vi "SS2 Live_Init FPGA.vi"(6 "Live Mode":bool, 8 "Error In":errorcluster, 9 "Current Image Set":i32, 10 "FPGA bitfile Path":path=path "C:/Data on Delator/SwissSPAD2/Software  64bit/matlab_code_fast_var_gate_v2/bit_file/ss2_top.bit", 11 "SS2 Live Internal Variables in":T1={"okCFrontPanelDevices Refnum"=refnum, "Device Refnum"=refnum, "Display Image"=refnum, "# Live Images"=0, "relative s"=0.0, "# Image Sets"=0, "Message"="", "Current Image Set"=0, "# Datasets"=0, "Current Dataset"=0, "Live Mode"=FALSE, "Recording Mode"=FALSE, "Record Button"=refnum, "Live Button"=refnum, "SS2 Live Gate Data Q Name"="SS2 Live Gate Data Q", "Discard First Image"=FALSE, "Image Information"={"Save ROI Only"=FALSE, "Left"=0, "Top"=0, "Right"=0, "Bottom"=0, "Use Current ROI"=FALSE}, "Image Binning Options"={"Use Image Binning"=FALSE, "X Bin"=1, "Y Bin"=1}} {"Image Binning Options"."Y Bin" min=1; "Image Binning Options"."X Bin" min=1}) -> (0 "Error Out":errorcluster, 1 "# 8-bit Images per Set":u32, 2 "Buffer Size (#8-bit Images)":u32, 3 "SS2 Live Internal Variables out":T1={"okCFrontPanelDevices Refnum"=refnum, "Device Refnum"=refnum, "Display Image"=refnum, "# Live Images"=0, "relative s"=0.0, "# Image Sets"=0, "Message"="", "Current Image Set"=0, "# Datasets"=0, "Current Dataset"=0, "Live Mode"=FALSE, "Recording Mode"=FALSE, "Record Button"=refnum, "Live Button"=refnum, "SS2 Live Gate Data Q Name"="SS2 Live Gate Data Q", "Discard First Image"=FALSE, "Image Information"={"Save ROI Only"=FALSE, "Left"=0, "Top"=0, "Right"=0, "Bottom"=0, "Use Current ROI"=FALSE}, "Image Binning Options"={"Use Image Binning"=FALSE, "X Bin"=1, "Y Bin"=1}} {"Image Binning Options"."Y Bin" min=1; "Image Binning Options"."X Bin" min=1})   [LabVIEW 2019]
uses:
  SS2 Live Internal Variables.ctl
  C:/UCLA Thinkpad Google Drive/LabVIEW 2019 SP1/builds/SS2 Live Distribution/Opal Kelly/C# Wrapper/libFrontPanel-csharp.dll
  Opal Kelly/C# Wrapper/libFrontPanel-csharp.dll
  <vilib>/vision/Image Controls.llb/IMAQ Image.ctl
  SS2 Live_Image ROI Information.ctl
  Phasor/Image Binning Options.ctl
  SS2 Live_Settings List.ctl
  Opal Kelly/C# Wrapper/okFrontPanelC#Wrapper.lvlib
  Variant/Variant to Data/Variant to Data.lvlib
panel:
  in  "milliseconds to wait":u32
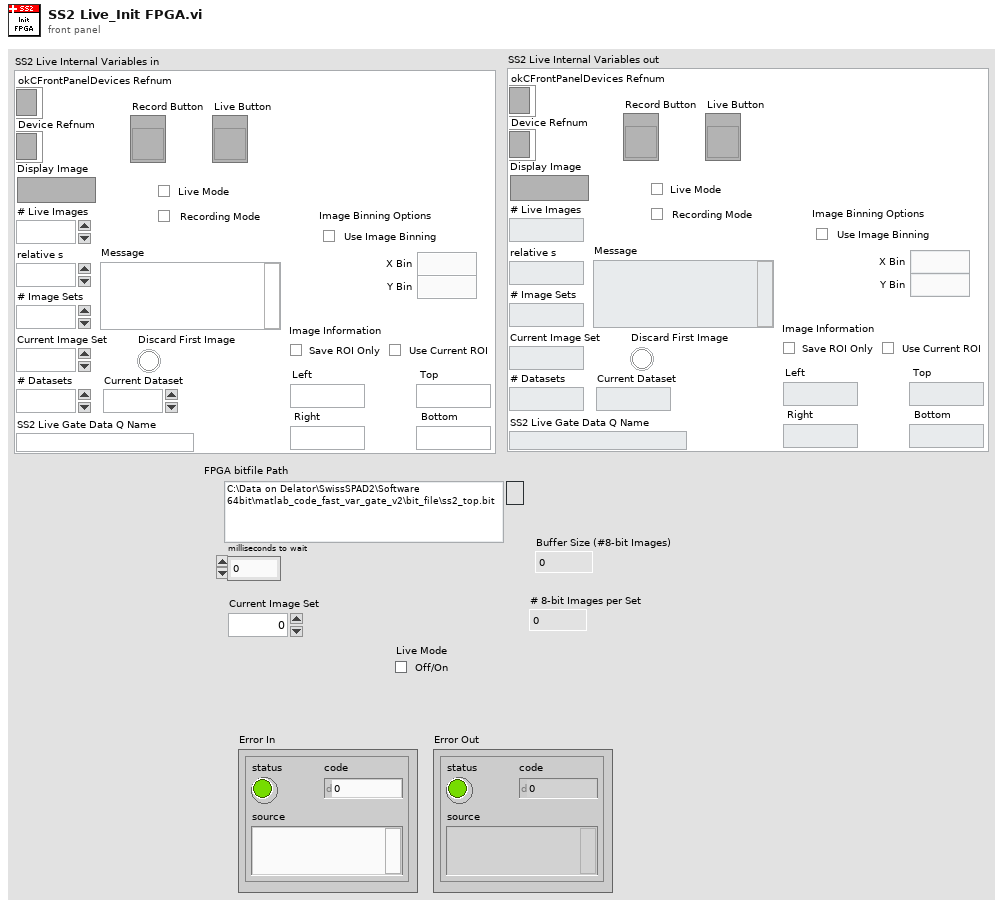
[diagram p1: front panel]
types:
  T1 = typedef "SS2 Live Internal Variables.ctl" = cluster{"okCFrontPanelDevices Refnum":refnum<k24>, "Device Refnum":refnum<k24>, "Display Image":T2, "# Live Images":i32, "relative s":dbl, "# Image Sets":i32, "Message":string, "Current Image Set":i32, "# Datasets":i32, "Current Dataset":i32, "Live Mode":bool, "Recording Mode":bool, "Record Button":refnum<vi>, "Live Button":refnum<vi>, "SS2 Live Gate Data Q Name":string, "Discard First Image":bool, "Image Information":T3, "Image Binning Options":T4}
  T2 = typedef "IMAQ Image.ctl" = refnum<image>
  T3 = typedef "SS2 Live_Image ROI Information.ctl" = cluster{"Save ROI Only":bool, "Left":u16, "Top":u16, "Right":u16, "Bottom":u16, "Use Current ROI":bool}
  T4 = typedef "Image Binning Options.ctl" = cluster{"Use Image Binning":bool, "X Bin":i32, "Y Bin":i32}
  T5 = typedef "SS2 Live_Settings List.ctl" = enum16{"FPGA:Bitfile Path", "FPGA:Bitfile Version", "Acquisition Parameters:SS2 DAQ Parameters", "Acquisition Parameters:Gate Configuration Array", "Acquisition Parameters:Buffer Size (# Gates)", "File Information:File Information", "File Information:# Datasets in Series", "Image Parameters:Image ROI Information", "Image Parameters:Image Binning Options", "UI Parameters:Histogram Bins Number"}
  T6 = typedef "SS2 DAQ Parameters 2.ctl" = cluster{"10 bits":bool, "# Exposure Sequences":u32, "# 1-bit Frame per Gate":u32, "Gate Shift":u32, "# Gates per Set":u32, "# Sets":u32, "Laser Period":dbl[unit], "Gate Offset":u32, "Auto-adjust Gate Offset":bool, "Gate Definition":T7}
  T7 = typedef "SS2 Gate Definition.ctl" = cluster{"gs_psincdec_0":u32, "gs_psincdec_1":u32, "gs_psincdec_2":u32, "gs_psincdec_3":u32, "gs_no_shift_adj_1":u32, "gs_no_shift_adj_2":u32, "gs_no_shift_adj_3":u32}
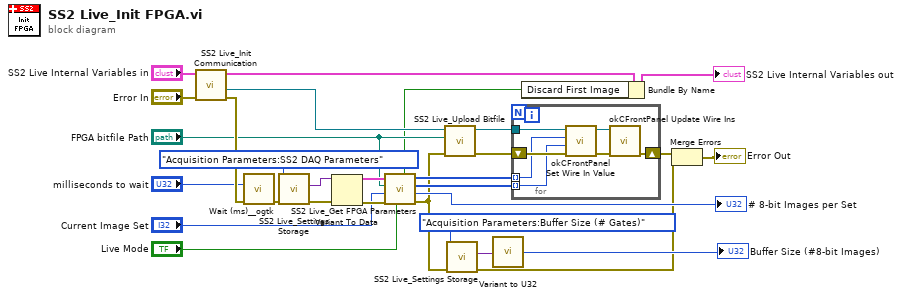
[diagram p0: block diagram]
diagram:
  n1 = call "SS2 Live_Init Communication.vi"("Error In"="Error In", "SS2 Live Internal Variables in"="SS2 Live Internal Variables in") -> ("Error Out"=w23:errorcluster, "Device Refnum"=w10:refnum<k24>, "SS2 Live Internal Variables out"=w9:T1)  [unwired: 6 in, 1 out]
  n2 = call <userlib>:"Wait (ms)__ogtk.vi"("error in (no error)"=w23, "milliseconds to wait"="milliseconds to wait") -> ("error out"=w13:errorcluster)  [unwired: 8 in, 1 out]
  n3 = call "SS2 Live_Settings Storage.vi"("Error In"=w13, "Settings List"=SS2_Live_Settings_List."Acquisition Parameters:SS2 DAQ Parameters") -> ("Error Out"=w20:errorcluster, "Variant Data out"=w21:variant)  [unwired: 8 in]
  n4 = Variant To Data(error in=w20, Variant=w21) -> (data=w17:T6, error out=w19:errorcluster)  [unwired: 1 in]
  n5 = call "SS2 Live_Get FPGA Parameters.vi"("Live Mode"="Live Mode", "Error In"=w19, "Current Image Set"="Current Image Set", "Bifile Path"="FPGA bitfile Path", "SS2 DAQ Parameters"=w17) -> ("Error Out"=w6:errorcluster, "#8-bit Images per Set"=→"# 8-bit Images per Set":u32, "SS2 FPGA DAQ Parameters"=w25:u32[], "SS2 FPGA DAQ Addresses"=w24:i32[], "Discard First Image"=w7:bool)  [unwired: 2 in]
  n6 = call "SS2 Live_Upload Bitfile.vi"("error in (no error)"=w6, "FPGA bitfile Path"="FPGA bitfile Path", "okCFrontPanel Device Refnum"=w10) -> ("error out"=w28:errorcluster, "okCFrontPanel Device Refnum"=w27:refnum<k24>)  [unwired: 7 in]
  n7 = call "SS2 Live_Settings Storage.vi"("Error In"=w6, "Settings List"=SS2_Live_Settings_List."Acquisition Parameters:Buffer Size (# Gates)") -> ("Error Out"=w1:errorcluster, "Variant Data out"=w4:variant)  [unwired: 8 in]
  n8 = call "Variant to U32.vi"("Variant"=w4) -> ("Value"=→"Buffer Size (#8-bit Images)":u32)  [unwired: 8 in]
  n9 = for {
    shift-right: [w31] -> w26
    shift-left: w28 -> [w36]
    tunnel: w25 -> [w34] mode=indexing
    tunnel: w24 -> [w30] mode=indexing
    tunnel: w27 -> [w35]
    n10 = call "okCFrontPanel Set Wire In Value.vi"("Error In"=w36, "Value"=w34, "Endpoint"=w30, "okCFrontPanel Refnum"=w35) -> ("Error Out"=w33:errorcluster, "okCFrontPanel Refnum"=w32:refnum<k24>)  [unwired: 6 in]
    n11 = call "okCFrontPanel Update Wire Ins.vi"("Error In"=w33, "okCFrontPanel Refnum"=w32) -> ("Error Out"=w31:errorcluster)  [unwired: 8 in, 1 out]
  }
  n12 = Bundle By Name(cluster=w9, "Discard First Image"=w7) -> (→"SS2 Live Internal Variables out":T1)
  n13 = Merge Errors(w26, w1) -> (→"Error Out":errorcluster)
